vi "Write Active.vi"(8 "error in (no error)":errorcluster, 10 "Active":bool, 11 "TTLController in":refnum<class "TTLController.lvclass">) -> (0 "error out":errorcluster, 3 "TTLController out":refnum<class "TTLController.lvclass">)   [LabVIEW 2020, in "TTLController.lvclass"]
uses:
  TTLController.lvclass
  TTLController.lvclass/TTLController.ctl
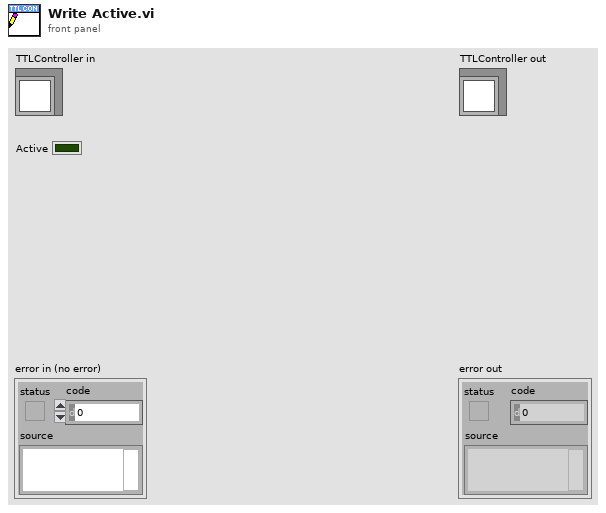
[diagram p1: front panel]
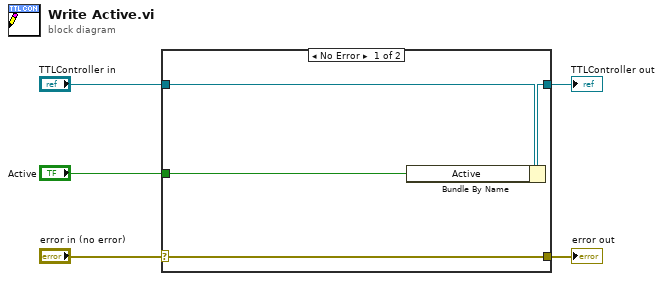
[diagram p0: block diagram]
diagram:
  n1 = case shown="No Error" "error in (no error)" {
    selector: "error in (no error)" -> [w9 w10]
    tunnel: [w9 w10] -> w4
    tunnel: [w7 w11] -> w2
    tunnel: "TTLController in" -> [w8 w11]
    tunnel: "Active" -> [w6 _]
    frame No Error {
      n2 = Bundle By Name(cluster=w8, "Active"=w6) -> (w7:refnum<class "TTLController.lvclass">)
    }
    frame Error {
    }
  }
  "error out" <- w4
  "TTLController out" <- w2
